vi "INI read mmWave adapters.vi"(8 "error in (no error)":T1) -> (0 "error out":T1, 2 "RX_adapter":string, 3 "TX_adapter":string)   [LabVIEW 2019, in "Shared.lvlib"]
uses:
  Shared.lvlib
  System GV.vi
  <vilib>/Utility/error.llb/Error Cluster From Error Code.vi
  <vilib>/ErrorRing/Error Ring.xnode
  <vilib>/Utility/config.llb/NI_LVConfig.lvlib
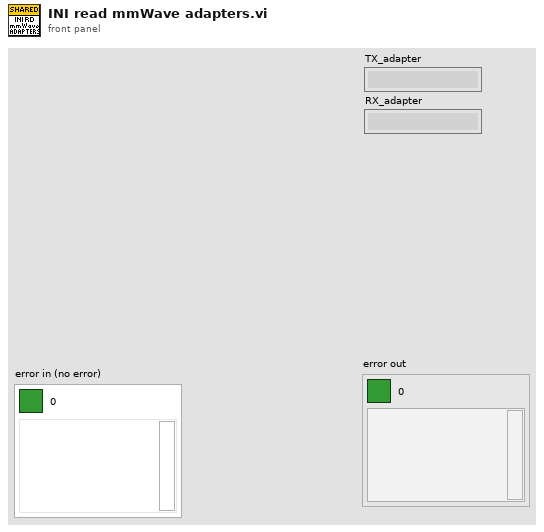
[diagram p1: front panel]
types:
  T1 = cluster{"Boolean Round":bool, "code":i32, "source":string}
  T2 = cluster{"TX_adapter":string, "RX_adapter":string}
  T3 = typedef "NI_LVConfig.lvlib/Config Data RefNum.ctl" = refnum<k1>
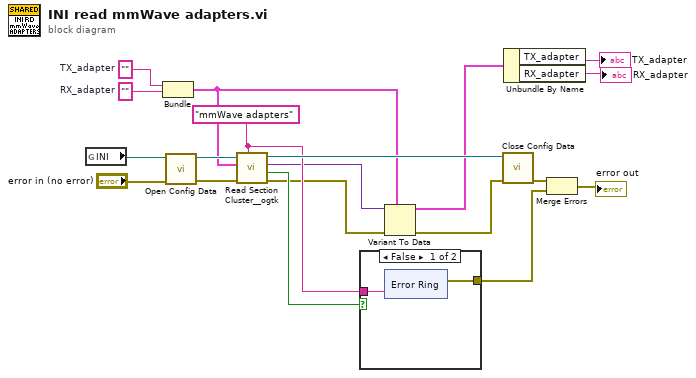
[diagram p0: block diagram]
diagram:
  w7 = ""  # RX_adapter
  w15 = ""  # TX_adapter
  w13 = "mmWave adapters" ("section (optional)")
  n1 = global read "System GV.vi" "INI"() -> (w16:path)
  n2 = Bundle("TX_adapter"=w15, "RX_adapter"=w7) -> (w9:T2)  [unwired: 1 in]
  n3 = call <vilib>:"Open Config Data.vi"("error in (no error)"="error in (no error)", "configuration file path"=w16) -> ("error out"=w17:errorcluster, "refnum"=w19:T3)  [unwired: 7 in, 1 out]
  n4 = call <userlib>:"Read Section Cluster__ogtk.vi"("section (optional)"=w13, "error in (no error)"=w17, "Section Formatted Cluster Type"=w9, "refnum"=w19) -> ("error out"=w11:errorcluster, "all found?"=w14:bool, "Section Formatted Cluster"=w12:variant, "dup refnum"=w18:T3)  [unwired: 3 in, 1 out]
  n5 = case shown="False" w14 {
    tunnel: w13 -> [w21 _]
    tunnel: [w20 _] -> w3
    frame False {
      n6 = xnode "Error Ring"("parameter 0"=w21) -> ("error out"=w20:errorcluster)
    }
    frame True {
    }
  }
  n7 = Variant To Data(error in=w11, type=w9, Variant=w12) -> (data=w8:T2, error out=w10:errorcluster)
  n8 = call <vilib>:"Close Config Data.vi"("error in (no error)"=w10, "refnum"=w18) -> ("error out"=w4:errorcluster)  [unwired: 8 in, 1 out]
  n9 = Unbundle By Name(w8) -> ("TX_adapter"=→"TX_adapter":string, "RX_adapter"=→"RX_adapter":string)
  n10 = Merge Errors(w4, w3) -> (→"error out":errorcluster)
